vi "Bundle Script_Set Property Node Items.vi"(8 "error in":errorcluster, 10 "Property Array":T1(array[cluster]), 11 "Property Node Ref":refnum<vi>) -> (0 "error out":errorcluster)   [LabVIEW 2023]
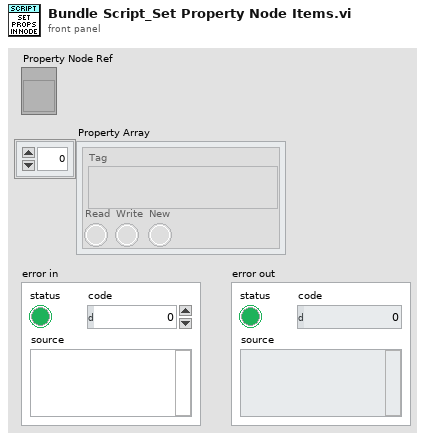
[diagram p1: front panel]
types:
  T1 = cluster{"Tag":string, "Read":bool, "Write":bool, "New":bool}[]
  T2 = cluster{"Index":u16, "Property Type":enum16{"Unknown", "Base", "Scripting", "Private", "Deprecated", "None", "Divider"}, "ID String":string, "Dotted ID String":string, "Class":string, "Parent":string, "Display name full":string, "Display name short":string, "Parents Array":string[], "Indent":u16}
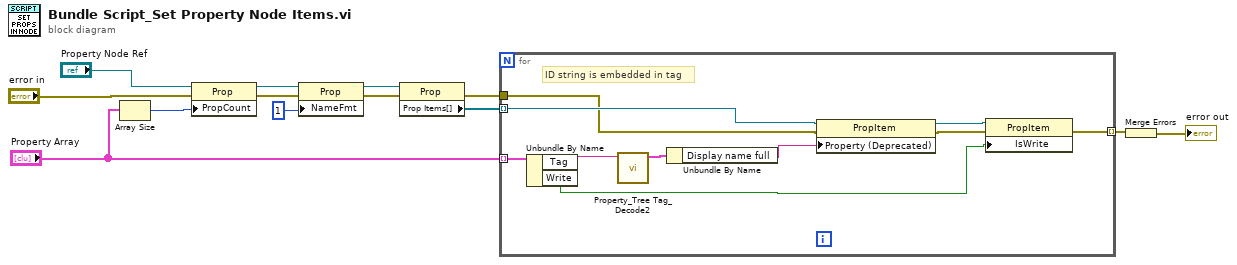
[diagram p0: block diagram]
diagram:
  n1 = Array Size(array="Property Array") -> (size(s)=w12:i32)
  n2 = property class="Prop"(reference="Property Node Ref", error in="error in", "PropCount"=w12) -> (reference out=w5:refnum<vi>, error out=w4:errorcluster)
  n3 = property class="Prop"(reference=w5, error in=w4, "NameFmt"=u32 1 ("Name Format")) -> (reference out=w3:refnum<vi>, error out=w2:errorcluster)
  n4 = property class="Prop"(reference=w3, error in=w2) -> (error out=w13:errorcluster, "Prop Items[]"=w7:refnum<vi>[])  [unwired: 1 out]
  n5 = for {
    tunnel: w7 -> [w18] mode=indexing
    tunnel: "Property Array" -> [w23] mode=indexing
    tunnel: [w21] -> w9 mode=indexing
    tunnel: w13 -> [w16]
    # "ID string is embedded in tag"
    n6 = Unbundle By Name(w23) -> ("Tag"=w19:string, "Write"=w22:bool)
    n7 = call "Property_Tree Tag_Decode2.vi"("Tag In"=w19) -> ("TagData"=w20:T2)  [unwired: 10 in]
    n8 = Unbundle By Name(w20) -> ("Display name full"=w17:string)
    n9 = property class="PropItem"(reference=w18, error in=w16, "Property (Deprecated)"=w17) -> (reference out=w14:refnum<vi>, error out=w15:errorcluster)
    n10 = property class="PropItem"(reference=w14, error in=w15, "IsWrite"=w22) -> (error out=w21:errorcluster)  [unwired: 1 out]
  }
  n11 = Merge Errors(w9) -> (→"error out":errorcluster)
